vi "18.2-DAQ-Asist-ContinuousVoltageIn.vi"() -> ()   [LabVIEW 2020]
doc: "This example demonstrates how to continuously acquire buffered voltage measurements using a DAQmx device.\n\nFor instructions on how to connect your signals to the DAQ device, refer to your device documentation."
panel:
  in  "Stop":bool
  out "Waveform Graph":dynamicdata(graph)
  # "Acquired Data"
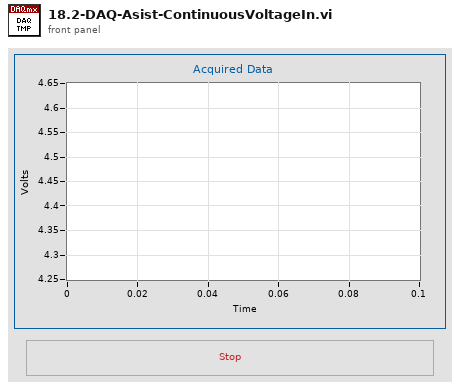
[diagram p1: front panel]
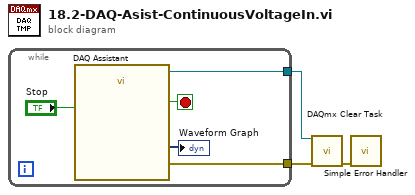
[diagram p0: block diagram]
diagram:
  n1 = while {
    tunnel: [w7] -> w3
    tunnel: [w6] -> w2
    stop <- w8 stop-if-true
    n2 = call "DAQ Assistant"("stop (F)"="Stop") -> ("task out"=w7:refnum<k21>, "data"=→"Waveform Graph":dynamicdata, "stopped"=w8:bool, "error out"=w6:errorcluster)  [unwired: 15 in]
  }
  n3 = call <vilib>:"DAQmx Clear Task.vi"("task in"=w3, "error in"=w2) -> ("error out"=w1:errorcluster)  [unwired: 13 in]
  n4 = call <vilib>:"Simple Error Handler.vi"("error in (no error)"=w1) -> ()  [unwired: 4 in, 5 out]
